vi "IIC Slave Write Remain.vi"(10 "IICIndex":i32, 11 "DevHandle":i32) -> (3 "function return":i32)   [LabVIEW 2010, in "usb2iic.lvlib"]
doc: "int WINAPI IIC_SlaveWriteRemain(int DevHandle,int IICIndex);"
uses:
  usb2iic.lvlib
  USB2XXX.dll
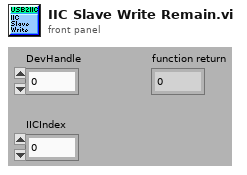
[diagram p1: front panel]
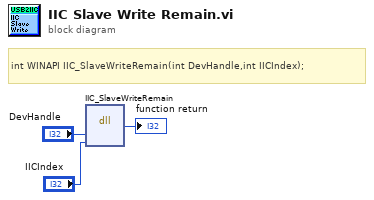
[diagram p0: block diagram]
diagram:
  # "int WINAPI IIC_SlaveWriteRemain(int DevHandle,int IICIndex);"
  n1 = dll-call lib="G:/OtherWork/USB2XXX_Example/trunk/Labview/PublicFiles/USB2XXX.*" fn="IIC_SlaveWriteRemain"("DevHandle"="DevHandle", "IICIndex"="IICIndex") -> (→"function return":i32)  [unwired: 5 in, 2 out]
